vi "Close.vi"(8 "error in (no error)":errorcluster, 11 "refnum":T1) -> (0 "error out":errorcluster)   [LabVIEW 2025, in "xTest.lvlib"]
uses:
  xTest.lvlib
  ContextProxy.ctl
  D:/xTestPlatform/xTestPlatform/bin/x86/Debug/net8.0-windows/win-x86/xTestPlatform.Interop.dll
  xTestPlatform/bin/x86/Debug/net8.0-windows/win-x86/xTestPlatform.Interop.dll
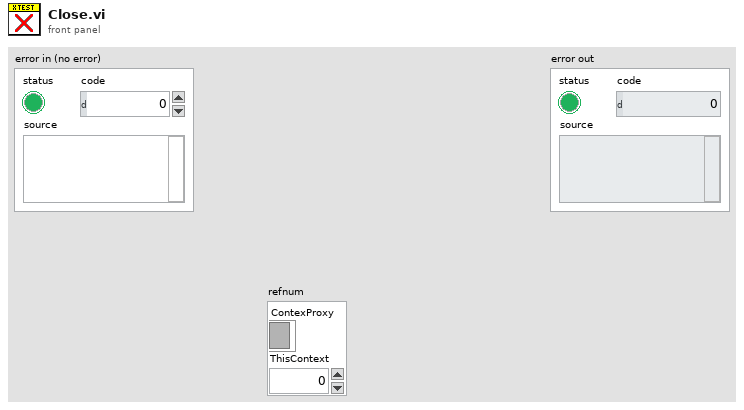
[diagram p1: front panel]
types:
  T1 = typedef "xTest.lvlib/ContextProxy.ctl" = cluster{"ContexProxy":refnum<k39>, "ThisContext":i32}
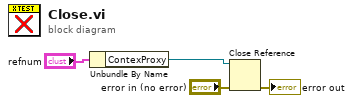
[diagram p0: block diagram]
diagram:
  n1 = Unbundle By Name("refnum") -> ("ContexProxy"=w3:refnum<k39>)
  n2 = Close Reference(reference=w3, error in (no error)="error in (no error)") -> (error out=→"error out":errorcluster)
